vi "Untitled 2.vi"() -> ()   [LabVIEW 2016]
uses:
  <vilib>/Utility/config.llb/Write Key (String).vi
  <vilib>/Utility/config.llb/Write Key (Boolean).vi
  <vilib>/Utility/config.llb/NI_LVConfig.lvlib
panel:
  in  "encoder direction":bool=TRUE
  in  "encoder":dbl format="%#_13g"
  in  "A":dbl format="%#_13g"
  in  "V":dbl format="%#_13g"
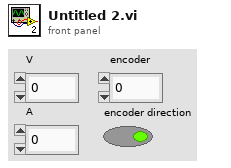
[diagram p1: front panel]
types:
  T1 = typedef "NI_LVConfig.lvlib/Config Data RefNum.ctl" = refnum<k1>
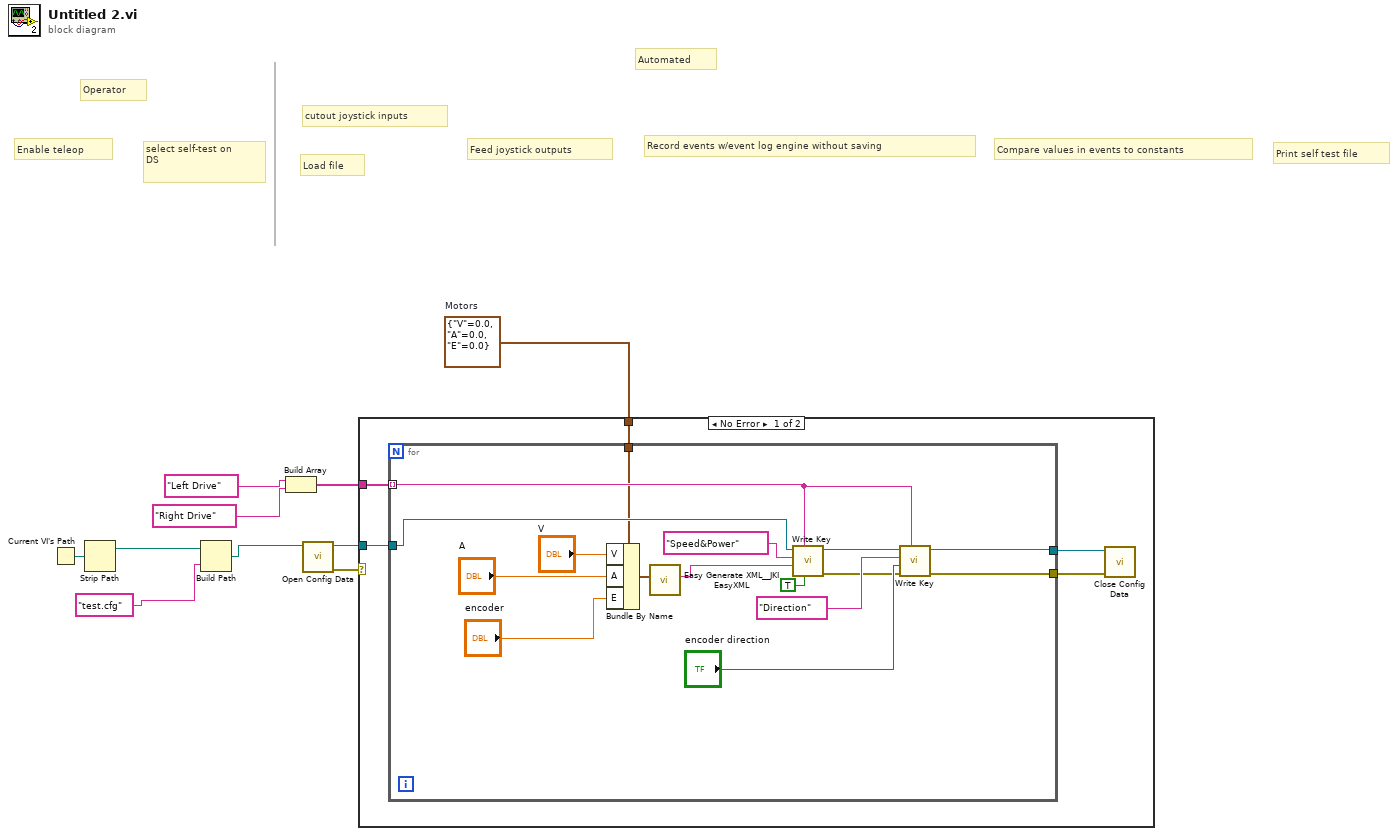
[diagram p0: block diagram]
diagram:
  w5 = cluster{"V":dbl, "A":dbl, "E":dbl} {"V"=0.0, "A"=0.0, "E"=0.0}  # Motors
  # "Automated"
  # "Operator"
  # "select self-test on\nDS"
  # "Enable teleop"
  # "Print self test file"
  # "Compare values in events to constants"
  # "Record events w/event log engine without saving"
  # "Feed joystick outputs"
  # "cutout joystick inputs"
  # "Load file"
  n1 = Current VI's Path() -> (path=w4:path)
  n2 = Strip Path(path=w4) -> (stripped path=w3:path)  [unwired: 1 out]
  n3 = Build Path(base path=w3, name or relative path="test.cfg") -> (appended path=w2:path)
  n4 = Build Array("Left Drive" ("key"), "Right Drive" ("key")) -> (w6:string[])
  n5 = call <vilib>:"Open Config Data.vi"("configuration file path"=w2) -> ("error out"=w9:errorcluster, "refnum"=w10:T1)  [unwired: 8 in, 1 out]
  n6 = case shown="No Error" w9 {
    tunnel: w10 -> [w15 _]
    tunnel: w6 -> [w13 _]
    tunnel: w5 -> [w12 _]
    frame No Error {
      n7 = for {
        tunnel: w15 -> [w26]
        tunnel: [w19] -> w14
        tunnel: w13 -> [w23] mode=indexing
        tunnel: w12 -> [w21]
        tunnel: [w18] -> w11
        n8 = Bundle By Name(cluster=w21, "V"="V", "A"="A", "E"="encoder") -> (w31:cluster{"V":dbl, "A":dbl, "E":dbl})
        n9 = call <vilib>:"Easy Generate XML__JKI EasyXML.vi"("LabVIEW Data"=w31) -> ("XML String"=w27:string)  [unwired: 9 in, 1 out]
        n10 = call-poly <vilib>:"Write Key.vi"("write raw string? (F)"=TRUE, "section"=w23, "value"=w27, "key"="Speed&Power" ("section"), "refnum"=w26) -> ("error out"=w17:errorcluster, "refnum out"=w25:T1)  [unwired: 4 in, 1 out]
        n11 = call-poly <vilib>:"Write Key.vi"("section"=w23, "error in (no error)"=w17, "value"="encoder direction", "key"="Direction", "refnum"=w25) -> ("error out"=w18:errorcluster, "refnum out"=w19:T1)  [unwired: 4 in, 1 out]
      }
      n12 = call <vilib>:"Close Config Data.vi"("error in (no error)"=w11, "refnum"=w14) -> ()  [unwired: 8 in, 2 out]
    }
    frame Error {
    }
  }
